vi "Convert Fractional Texel To Index.vi"(11 "Texel Start":T1) -> (3 "Texel As Pixel":T2)   [LabVIEW 2022 SP3, in "Raster.lvlib"]
uses:
  Raster.lvlib
  Point 2D (I32).ctl
  Point 2D (SGL).ctl
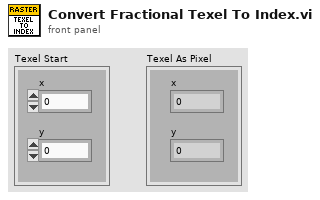
[diagram p1: front panel]
types:
  T1 = typedef "Raster.lvlib/Point 2D (SGL).ctl" = cluster{"x":sgl, "y":sgl}
  T2 = typedef "Raster.lvlib/Point 2D (I32).ctl" = cluster{"x":i32, "y":i32}
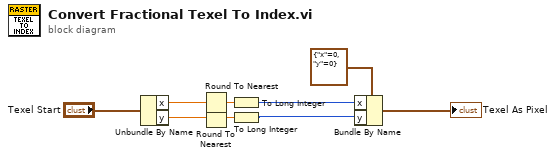
[diagram p0: block diagram]
diagram:
  n1 = Unbundle By Name("Texel Start") -> ("x"=w5:sgl, "y"=w2:sgl)
  n2 = Round To Nearest(number=w5) -> (nearest integer value=w6:sgl)
  n3 = Round To Nearest(number=w2) -> (nearest integer value=w3:sgl)
  n4 = To Long Integer(number=w6) -> (32bit integer=w4:i32)
  n5 = To Long Integer(number=w3) -> (32bit integer=w1:i32)
  n6 = Bundle By Name(cluster=T2 {"x"=0, "y"=0} ("Point"), "x"=w4, "y"=w1) -> (→"Texel As Pixel":T2)
